vi "Destructor.vi"(8 "error  in":errorcluster, 11 "SerDes in":refnum<class "OOPbyRef.lvclass">) -> (0 "error out":errorcluster, 3 "SerDes out":refnum<class "OOPbyRef.lvclass">)   [LabVIEW 2021, in "DQMH_byOOPRef.lvlib" / "OOPbyRef.lvclass"]
doc: "<b>Note:</b> This VI was modified by the <b>Validate DQMH Module</b> tool to be shared clone reentrant."
uses:
  OOPbyRef.lvclass
  OOPbyRef.lvclass/OOPbyRef.ctl
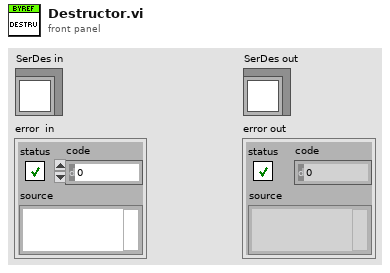
[diagram p1: front panel]
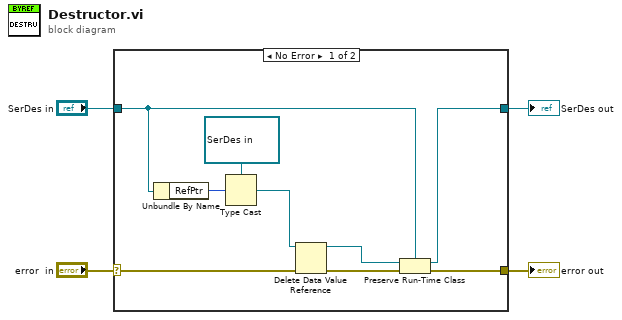
[diagram p0: block diagram]
diagram:
  n1 = case shown="No Error" "error  in" {
    selector: "error  in" -> [w10 w15]
    tunnel: [w7 w15] -> w3
    tunnel: [w5 w14] -> w1
    tunnel: "SerDes in" -> [w6 w14]
    frame No Error {
      n2 = Unbundle By Name(w6) -> ("RefPtr"=w13:i32)
      n3 = Type Cast(type=refnum<data-value> refnum ("data value reference"), x=w13) -> (*(type *) &x=w11:refnum<data-value>)
      n4 = Delete Data Value Reference(data value reference=w11, error in=w10) -> (data value=w9:refnum<class "OOPbyRef.lvclass">, error out=w8:errorcluster)
      n5 = Preserve Run-Time Class(object in=w9, error in=w8, 2:w6) -> (object out=w5:refnum<class "OOPbyRef.lvclass">, error out=w7:errorcluster)
    }
    frame Error {
    }
  }
  "error out" <- w3
  "SerDes out" <- w1
